vi "Paths Sub-Parser.vi"(0 "XML File Path In":path, 2 "error in (no error)":errorcluster) -> (3 "XML File Path Out":path, 4 "paths":T2(array[cluster]), 5 "funnels":T2(array[cluster]), 6 "error out":errorcluster)   [LabVIEW 2016]
doc: "This VI takes an array of XML path nodes as input and uses LabVIEW's built-in XPath parser to pull out information about each path. Specifically, it gets the style ('style') and the path data ('d') and parses each one. Then it determines whether the path is actually a funnel and creates two arrays accordingly."
uses:
  <vilib>/Analysis/Matrix/Datatypes/RealMatrix.ctl
  <vilib>/Analysis/baseanly.llb/Real A x B.vi
  <vilib>/Analysis/NI_AALBase.lvlib
  <vilib>/Analysis/Matrix/NI_Matrix.lvlib
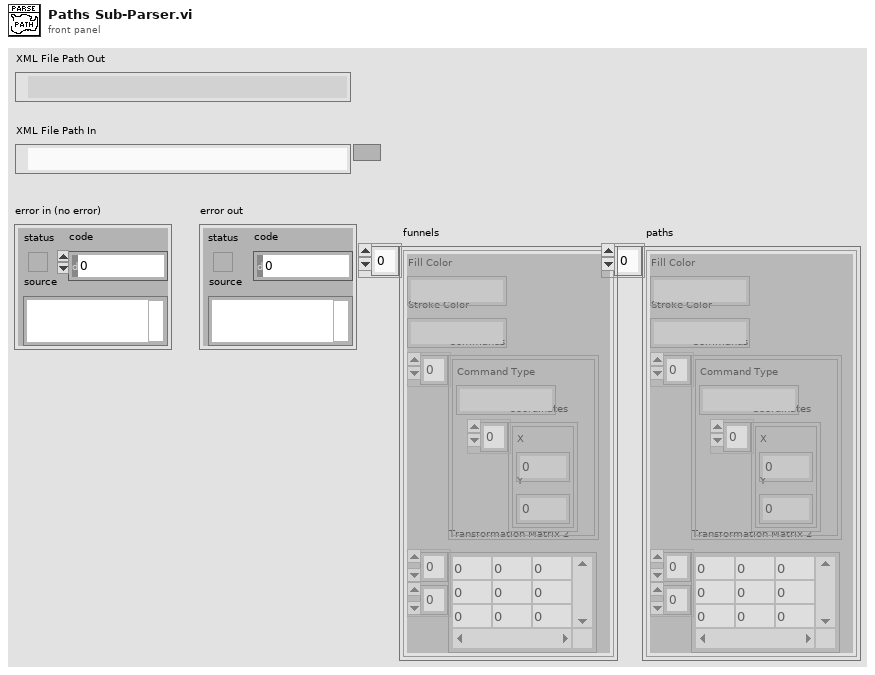
[diagram p1: front panel]
types:
  T1 = typedef "NI_Matrix.lvlib/RealMatrix.ctl" = dbl[][]
  T2 = cluster{"Fill Color":string, "Stroke Color":string, "Commands":cluster{"Command Type":string, "Coordinates":cluster{"X":dbl, "Y":dbl}[]}[], "Transformation Matrix 2":T1}[]
  T3 = cluster{"Command Type":string, "Coordinates":cluster{"X":dbl, "Y":dbl}[]}[]
  T4 = cluster{"Fill":string, "Stroke":string, "Commands":cluster{"Command Type":string, "Coordinates":cluster{"X":dbl, "Y":dbl}[]}[], "Transformation Matrix":T1}
  T5 = cluster{"Fill":string, "Stroke":string, "Commands":cluster{"Command Type":string, "Coordinates":cluster{"X":dbl, "Y":dbl}[]}[], "Transformation Matrix":T1}[]
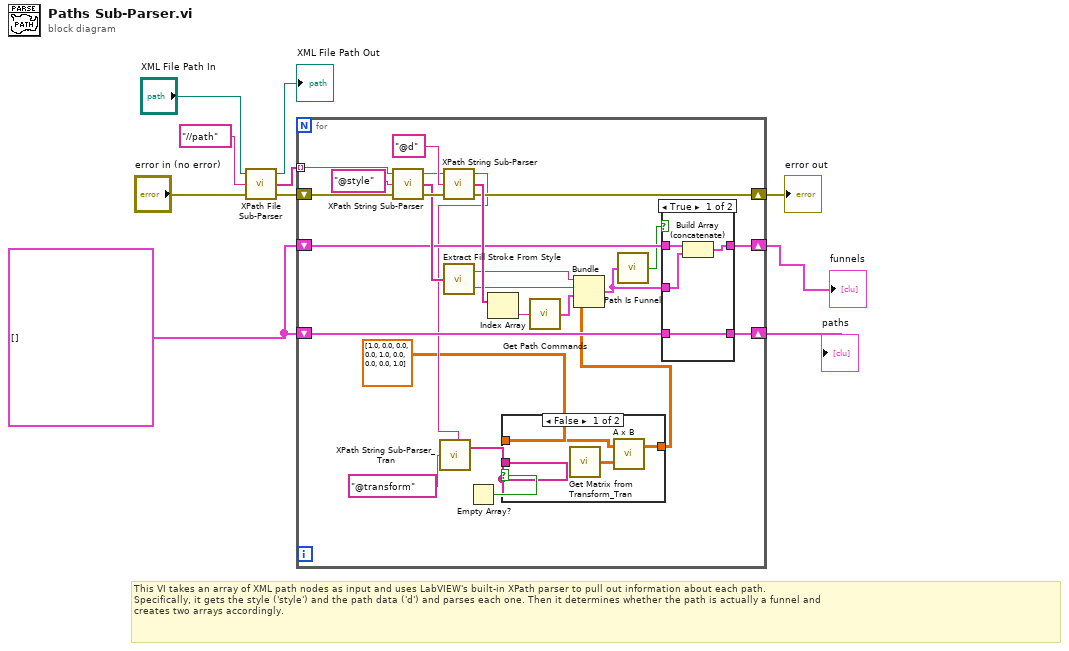
[diagram p0: block diagram]
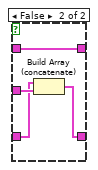
[diagram p3: hidden frame]
diagram:
  w2 = T2 [] ("paths 2")
  # "This VI takes an array of XML path nodes as input and uses LabVIEW's built-in XPath parser to pull out information about each path. \nSpecifically, it gets the style ('style') and the path data ('d') and parses each one. Then it determines whether the path is actually a funnel and\ncreates two arrays accordingly."
  n1 = call "XPath File Sub-Parser.vi"("error in (no error)"="error in (no error)", "XPath Expression"="//path" ("XPath expression"), "XML File Path In"="XML File Path In") -> ("error out"=w5:errorcluster, "Array of Results"=w7:string[], "XML File Path Out"=→"XML File Path Out":path)
  n2 = for {
    tunnel: w7 -> [w31] mode=indexing
    shift-right: [w24] -> w10
    shift-left: w5 -> [w34]
    shift-right: [w21] -> w9
    shift-left: w2 -> [w23]
    shift-right: [w19] -> w1
    shift-left: w2 -> [w22]
    n3 = call "XPath String Sub-Parser.vi"("error in (no error)"=w34, "XPath expression"="@style", "XML String In"=w31) -> ("error out"=w33:errorcluster, "Array of Results"=w26:string[], "XML String Out"=w25:string)
    n4 = call "XPath String Sub-Parser.vi"("error in (no error)"=w33, "XPath expression"="@d", "XML String In"=w25) -> ("error out"=w24:errorcluster, "Array of Results"=w30:string[], "XML String Out"=w15:string)
    n5 = call "XPath String Sub-Parser_Tran.vi"("XPath expression"="@transform", "XML String"=w15) -> ("Array of Results"=w12:string[])  [unwired: 1 in, 1 out]
    n6 = call "Extract Fill Stroke From Style.vi"("Array of Results"=w26) -> ("Fill"=w27:string, "Stroke"=w28:string)
    n7 = Empty Array?(array=w12) -> (empty?=w13:bool)
    n8 = Index Array(array=w30) -> (element=w29:string)  [unwired: 1 in]
    n9 = case shown="False" w13 {
      tunnel: [w39 w40] -> w11
      tunnel: w12 -> [w37 _]
      tunnel: T1 [[1.0, 0.0, 0.0], [0.0, 1.0, 0.0], [0.0, 0.0, 1.0]] ("Transformation Matrix") -> [w36 w40]
      frame False {
        n10 = call "Get Matrix from Transform_Tran.vi"("Transform Attributes"=w37) -> ("Matrix"=w38:T1)
        n11 = call-poly <vilib>:"A x B.vi"("B"=w38, "A"=w36) -> ("A x B"=w39:T1)  [unwired: 1 out]
      }
      frame True {
      }
    }
    n12 = call "Get Path Commands.vi"("Commands Raw Data"=w29) -> ("Commands"=w20:T3)
    n13 = Bundle("Fill"=w27, "Stroke"=w28, "Commands"=w20, "Transformation Matrix"=w11) -> (w17:T4)  [unwired: 1 in]
    n14 = call "Path Is Funnel.vi"("Path Information"=w17) -> ("Is Funnel?"=w18:bool)
    n15 = case shown="True" w18 {
      tunnel: w23 -> [w44 w46]
      tunnel: w22 -> [w43 w48]
      tunnel: [w44 w45] -> w21
      tunnel: w17 -> [w42 w47]
      tunnel: [w41 w48] -> w19
      frame True {
        n16 = Build Array (concatenate)(w43, w42) -> (w41:T5)
      }
      frame False {
        n17 = Build Array (concatenate)(w46, w47) -> (w45:T5)
      }
    }
  }
  "error out" <- w10
  "funnels" <- w1
  "paths" <- w9
